vi "DrivePath.vi"() -> ()   [LabVIEW 2018]
uses:
  Framework/Robot Global Data.vi
panel:
  in  "PathFileName":string
  in  "Index":dbl
  in  "NoWait":bool
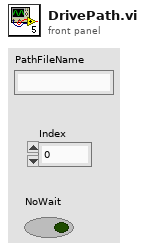
[diagram p1: front panel]
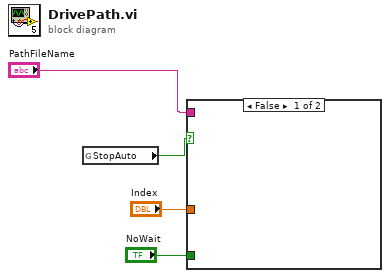
[diagram p0: block diagram]
diagram:
  n1 = global read "Robot Global Data.vi" "StopAuto"() -> (w4:bool)
  n2 = case shown="False" w4 {
    tunnel: "Index" -> [_ _]
    tunnel: "NoWait" -> [_ _]
    tunnel: "PathFileName" -> [_ _]
    frame False {
    }
    frame True {
    }
  }
